vi "Counter_SetPulseWidth.vi"(4 "error in (no error)":errorcluster, 5 "low period":dbl, 6 "high period":dbl, 7 "Task ID":u32) -> (0 "error out":errorcluster, 3 "Task ID":u32)   [LabVIEW 2015]
uses:
  Windows/System32/AdvLvDaq.dll
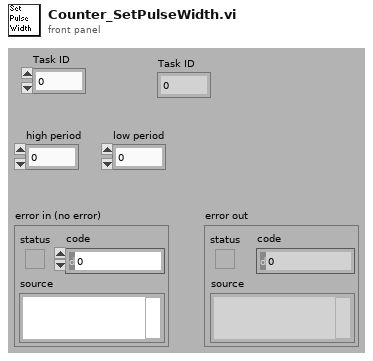
[diagram p1: front panel]
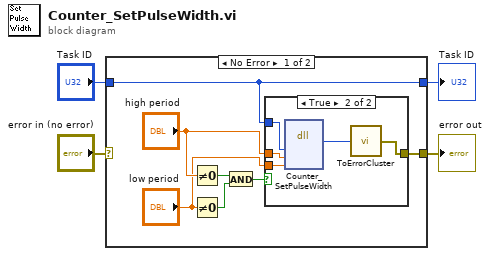
[diagram p0: block diagram]
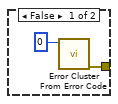
[diagram p2: hidden frame]
diagram:
  n1 = case shown="No Error" "error in (no error)" {
    selector: "error in (no error)" -> [_ w19]
    tunnel: "Task ID" -> [w5 w20]
    tunnel: [w6 w19] -> w2
    tunnel: [w5 w20] -> w1
    frame No Error {
      n2 = Not Equal To 0?(x="high period") -> (x != 0?=w11:bool)
      n3 = Not Equal To 0?(x="low period") -> (x != 0?=w10:bool)
      n4 = And(x=w11, y=w10) -> (x .and. y?=w9:bool)
      n5 = case shown="True" w9 {
        tunnel: w5 -> [_ w18]
        tunnel: "high period" -> [_ w17]
        tunnel: "low period" -> [_ w16]
        tunnel: [w13 w14] -> w6
        frame False {
          n6 = call <vilib>:"Error Cluster From Error Code.vi"("error code (0)"=0) -> ("error out"=w13:errorcluster)  [unwired: 2 in, 6 out]
        }
        frame True {
          n7 = dll-call lib="C:/Windows/System32/AdvLvDaq.dll" fn="Counter_SetPulseWidth"("taskId"=w18, "hiPeriod"=w17, "loPeriod"=w16) -> ("return type"=w15:i32)  [unwired: 6 in, 2 out]
          n8 = call "ToErrorCluster.vi"("error code"=w15) -> ("error out"=w14:errorcluster)
        }
      }
    }
    frame Error {
    }
  }
  "Task ID" <- w1
  "error out" <- w2
